vi "F8588A Test2.vi"() -> ()   [LabVIEW 2013]
uses:
  DMM/3458A Virtual Channel Config.ctl
  DMM/3458A Digitizing Low Levels/Configure/First Sample Trigger.ctl
  DMM/3458A Digitizer Session.ctl
  Counter/Counter Session.ctl
  Counter/Counter Type.ctl
  AWG/AWG Session.ctl
  AWG/AWG Type.ctl
  DMM/3458A Sync Mode.ctl
  DMM/3458A Idn Mode.ctl
  DMM/3458A Digitizing Low Levels/Configure/Sampling Mode.ctl
  DMM/3458A Digitizing Process Options.ctl
  DMM/3458A Data Packet.ctl
  DMM/3458A Aux Record Data.ctl
  DMM/3458A Digitizing Low Levels/Configure/Level Setup.ctl
  DMM/3458A Aperture Selection Mode.ctl
  DMM/3458A Multiplexing Config.ctl
  DMM/3458A Virtual Digitizer.lvlib
  Counter/Counter.lvlib
  AWG/AWG.lvlib
  DMM/3458A Digitizing Low Levels/3458A Digitizing Low Levels.lvlib
panel:
  in  "TRIG source (AUTO)":T1
  in  "samples count (100)":i32=100
  in  "apperture [s] (1.4 us)":dbl=1.4e-06 format="%#_6p"
  in  "sample period [s] (1 ms)":dbl=0.001 format="%#_6p"
  in  "channels":T2[](array[typedef])=[{"VISA"="GPIB0::11::INSTR", "Range [Vpk]"=10.0, "btn clr"=FALSE, "btn up"=FALSE, "btn down"=FALSE, "F8588"=TRUE}] {"Range [Vpk]" min=0.0}
  out "error out":errorcluster
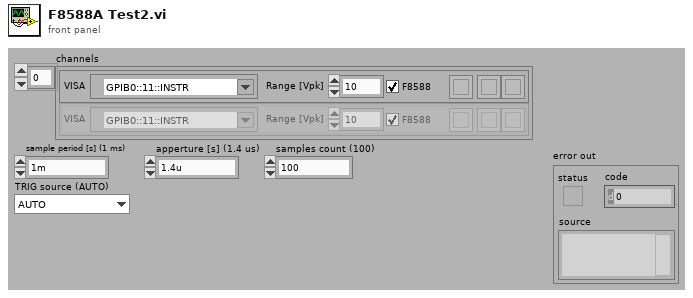
[diagram p1: front panel]
types:
  T1 = typedef "3458A Virtual Digitizer.lvlib/3458A Digitizing Low Levels.lvlib/First Sample Trigger.ctl" = enum16{"AUTO", "EXT", "SYN", "SGL", "HOLD", "LEVEL"}
  T2 = typedef "3458A Virtual Digitizer.lvlib/3458A Virtual Channel Config.ctl" = cluster{"VISA":refnum<visa-resource-name>, "Range [Vpk]":dbl, "btn clr":bool, "btn up":bool, "btn down":bool, "F8588":bool}
  T3 = typedef "3458A Virtual Digitizer.lvlib/3458A Digitizer Session.ctl" = cluster{"channels":T2[], "sync unit":T4, "awg unit":T6, "sync mode":T8, "streaming mode":bool, "idn mode":T9, "sampling mode":T10, "Ts [s]":dbl, "sample memory [B]":i32, "proc setup":T11, "sample size [B]":i32, "sample count":i32, "aux data":T13, "ranges [V]":dbl[], "aperture [s]":dbl, "LEVEL trigger":T14, "trigger mode":T1, "measure temp.?":bool, "disp mesages":string[], "shared bus?":bool, "disable display?":bool, "aper mode":T15, "aper rules":dbl[][], "multiplex":T16}
  T4 = typedef "Counter.lvlib/Counter Session.ctl" = cluster{"VISA":refnum<visa-resource-name>, "type":T5}
  T5 = typedef "Counter.lvlib/Counter Type.ctl" = enum16{"Picotest U6200A", "dummy"}
  T6 = typedef "AWG.lvlib/AWG Session.ctl" = cluster{"type":T7, "VISA":refnum<visa-resource-name>, "enable 10MHz ref":bool}
  T7 = typedef "AWG.lvlib/AWG Type.ctl" = enum16{"Agilent 331xxA to 332xxA", "Agilent 335xxA to 336xxA", "Tektronix AFG3101C", "dummy"}
  T8 = typedef "3458A Virtual Digitizer.lvlib/3458A Sync Mode.ctl" = enum16{"MASTER-SLAVE, MASTER clocked by TIMER", "MASTER-SLAVE, MASTER clocked by AWG", "ALL clocked by AWG", "MASTER-SLAVE, ALL clocked by TIMER", "ALL clocked by AWG with DFLL"}
  T9 = typedef "3458A Virtual Digitizer.lvlib/3458A Idn Mode.ctl" = enum16{"Auto", "Sequential (chn A, chn B, ...)", "From calibration string"}
  T10 = typedef "3458A Virtual Digitizer.lvlib/3458A Digitizing Low Levels.lvlib/Sampling Mode.ctl" = enum16{"DCV", "DSDC", "DSAC"}
  T11 = typedef "3458A Virtual Digitizer.lvlib/3458A Digitizing Process Options.ctl" = cluster{"channel id":i32, "packet size [smpl]":i32, "current timeout [s]":dbl, "blk2blk timeout [s]":dbl, "event time":timestamp, "stop notifier":refnum<notifier>, "data queues":refnum<queue>[], "proc refs":refnum<vi>[], "bus semaphore":T12}
  T12 = typedef "Semaphore RefNum" = refnum<k1>
  T13 = typedef "3458A Virtual Digitizer.lvlib/3458A Aux Record Data.ctl" = cluster{"channel id":i32, "valid?":bool[], "gain [V]":dbl[], "timestamp [s]":dbl[], "Ts [s]":dbl, "abs timestamp":timestamp, "t [deg C]":dbl[], "multiplex timestamp [s]":dbl, "only multiplex?":bool, "multiplex smpl offset":i64}
  T14 = typedef "3458A Virtual Digitizer.lvlib/3458A Digitizing Low Levels.lvlib/Level Setup.ctl" = cluster{"edge":enum16{"POS", "NEG"}, "level [V]":dbl, "coupling":enum16{"DC", "AC"}}
  T15 = typedef "3458A Virtual Digitizer.lvlib/3458A Aperture Selection Mode.ctl" = enum16{"Manual", "Maximum", "Table"}
  T16 = typedef "3458A Multiplexing Config.ctl" = cluster{"cycles":i32, "delay [s]":dbl, "enabled":bool, "overhead [s]":dbl, "tot smpls":i64, "sub-rec":i32, "overhead [%]":dbl}
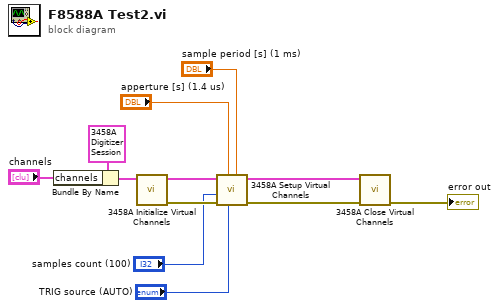
[diagram p0: block diagram]
diagram:
  n1 = Bundle By Name(cluster=T3 {"channels"=[{"VISA"="GPIB0::11::INSTR", "Range [Vpk]"=1.0, "btn clr"=FALSE, "btn up"=FALSE, "btn down"=FALSE, "F8588"=TRUE}], "sync unit"={"VISA"="", "type"=enum."Picotest U6200A"}, "awg unit"={"type"=enum."dummy", "VISA"="GPIB1::11::INSTR", "enable 10MHz ref"=TRUE}, "sync mode"=enum."MASTER-SLAVE, MASTER clocked by TIMER", "streaming mode"=TRUE, "idn mode"=enum."Auto", "sampling mode"=enum."DCV", "Ts [s]"=0.0001, "sample memory [B]"=135000000, "proc setup"={"channel id"=0, "packet size [smpl]"=64000, "current timeout [s]"=30.0, "blk2blk timeout [s]"=30.0, "event time"=timestamp(3467449553.84375 s since 1904-01-01), "stop notifier"=refnum, "data queues"=[refnum], "proc refs"=[refnum], "bus semaphore"=refnum}, "sample size [B]"=4, "sample count"=10000, "aux data"={"channel id"=0, "valid?"=[TRUE], "gain [V]"=[1.0], "timestamp [s]"=[0.0], "Ts [s]"=0.0001, "abs timestamp"=timestamp(3467449552.890625 s since 1904-01-01), "t [deg C]"=[nan], "multiplex timestamp [s]"=0.0, "only multiplex?"=FALSE, "multiplex smpl offset"=0}, "ranges [V]"=[1.0], "aperture [s]"=7e-05, "LEVEL trigger"={"edge"=enum."POS", "level [V]"=0.0, "coupling"=enum."DC"}, "trigger mode"=enum."LEVEL", "measure temp.?"=FALSE, "disp mesages"=["CHN-1"], "shared bus?"=FALSE, "disable display?"=FALSE, "aper mode"=enum."Table", "aper rules"=[[8000.0, 0.000102], [10000.0, 7e-05], [100000.0, 1.4e-06]], "multiplex"={"cycles"=2, "delay [s]"=0.2, "enabled"=FALSE, "overhead [s]"=0.5, "tot smpls"=10000, "sub-rec"=1, "overhead [%]"=1.0}} ("digitizer in"), "channels"="channels") -> (w12:T3)
  n2 = call "3458A Initialize Virtual Channels.vi"("digitizer in"=w12) -> ("error out"=w9:errorcluster, "digitizer out"=w8:T3)  [unwired: 6 in, 3 out]
  n3 = call "3458A Setup Virtual Channels.vi"("sample period [s] (1 ms)"="sample period [s] (1 ms)", "TRIG source (AUTO)"="TRIG source (AUTO)", "apperture [s] (1.4 us)"="apperture [s] (1.4 us)", "error in"=w9, "samples count (100)"="samples count (100)", "digitizer in"=w8) -> ("error out"=w3:errorcluster, "digitizer out"=w2:T3)  [unwired: 4 in]
  n4 = call "3458A Close Virtual Channels.vi"("error in"=w3, "session in"=w2) -> ("error out"=→"error out":errorcluster)  [unwired: 8 in, 1 out]
